vi "Denormalize Target.vi"(10 "Target In":T3, 11 "Image In":T2) -> (3 "Target Out":T1)   [LabVIEW 2015]
uses:
  <vilib>/vision/Image Controls.llb/IMAQ Image.ctl
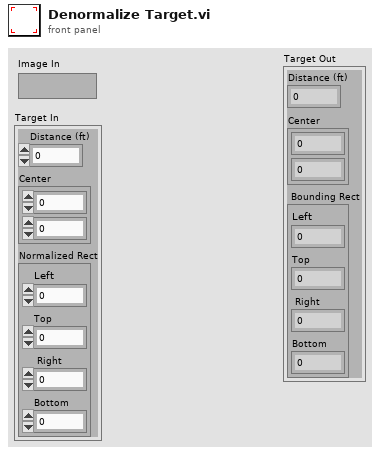
[diagram p1: front panel]
types:
  T1 = cluster{"Distance (ft)":dbl, "Center":cluster{dbl, dbl}, " Bounding Rect":cluster{"Left":dbl, "Top":dbl, " Right":dbl, "Bottom":dbl}}
  T2 = typedef "IMAQ Image.ctl" = refnum<image>
  T3 = cluster{"Distance (ft)":dbl, "Center":cluster{dbl, dbl}, "Normalized Rect":cluster{"Left":dbl, "Top":dbl, " Right":dbl, "Bottom":dbl}}
  T4 = cluster{"Left":dbl, "Top":dbl, " Right":dbl, "Bottom":dbl}
  T5 = cluster{"X Resolution":i32, i32, "X Resolution":i32, i32}
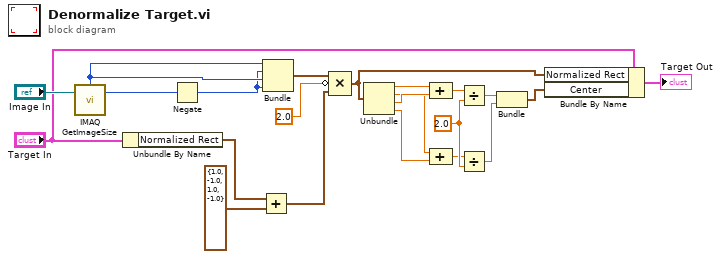
[diagram p0: block diagram]
diagram:
  w7 = 2.0
  n1 = call "IMAQ GetImageSize"("Image"="Image In") -> ("Y Resolution"=w12:i32, "X Resolution"=w21:i32)  [unwired: 3 in, 1 out]
  n2 = Unbundle By Name("Target In") -> ("Normalized Rect"=w15:T4)
  n3 = Negate(x=w12) -> (-x=w13:i32)
  n4 = Add(x=w15, y=cluster{dbl, dbl, dbl, dbl} {1.0, -1.0, 1.0, -1.0}) -> (x+y=w14:cluster{dbl, dbl, dbl, dbl})
  n5 = Bundle("X Resolution"=w21, w13, "X Resolution"=w21, w13) -> (w19:T5)  [unwired: 1 in]
  n6 = Compound Arithmetic op=MULTIPLY(w19, invert 2.0, w14) -> (w2:cluster{dbl, dbl, dbl, dbl})
  n7 = Unbundle(w2) -> (w11:dbl, w8:dbl, w10:dbl, w9:dbl)
  n8 = Compound Arithmetic op=ADD(w11, w10) -> (w6:dbl)
  n9 = Compound Arithmetic op=ADD(w8, w9) -> (w5:dbl)
  n10 = Divide(x=w6, y=w7) -> (x/y=w4:dbl)
  n11 = Divide(x=w5, y=w7) -> (x/y=w3:dbl)
  n12 = Bundle(w4, w3) -> (w1:cluster{dbl, dbl})  [unwired: 1 in]
  n13 = Bundle By Name(cluster="Target In", "Normalized Rect"=w2, "Center"=w1) -> (→"Target Out":T3)
